vi "FUG-HCN.GetRatedCurrent.vi"(0 "i ref in":refnum<vi>, 2 "Time out":i32, 5 "error in (no error)":errorcluster) -> (14 "i ref out":refnum<vi>, 16 "timed out":bool, 17 "Rated Current{mA}":dbl format="%.2f", 19 "error out":errorcluster)   [LabVIEW 2014, in "FUG-HCN.lvlib"]
doc: "Reads the rated current from the device."
uses:
  FUG-HCN.lvlib
  CSCore/CSSystem/CoreDefs/CoreDefs.error_type.ctl
  CSCore/CSSystem/CoreLib/CoreLib.lvlib
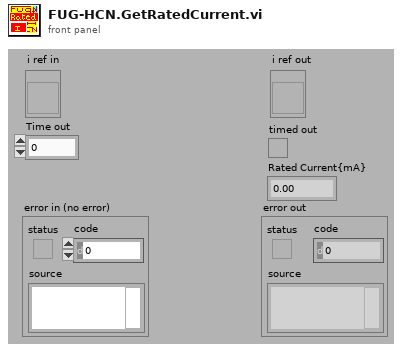
[diagram p1: front panel]
types:
  T1 = cluster{"VISA resource name":refnum<visa-resource-name>, "Gen time out":dbl, "timeout (0)":u32}
  T2 = typedef "CoreDefs.error_type.ctl" = enum16{"no error", "can't load process", "can't unload process", "process does not exist", "can't install process", "can't remove process", "unknown function", "time out", "can't execute function", "duplicate queue name", "super not found", "caller queue invalid", "can't ping process", "unknown error", "VISA Error", "VISA timeout", "GPIB timeout", "GPIB error", "communication error", "data type mismatch", "can't read data from OPC server", "can't write data to OPC server", "OET error", "function not implemented", "process already exists", "invalid Shared Variable name", "error writing Shared Variable", "error reading Shared Variable", "invalid client name", "corrupt database", "unknown class", "call not authorized", "parameter out of range", "OET timeout: can't get data to modify", "invalid queue name", "requested operation incompatible with current state", "event undefined", "event disabled", "state undefined", "caller is not a friend", "EventBuilder: bad eventID", "EventBuilder: no DAQ devices", "a thread must not stop itself", "UNUSED ELEMENT4", "DiscArchiver: eventData incomplete", "DiscArchiver: eventData does not belong to run", "DiscArchiver: can't open file", "DiscArchiver: can't write to file", "DiscArchiver: available disc space low", "can't acquire semaphore", "error reading data from database", "notifier object is not existing", "can't register process", "can't unregister process", "illegal event type", "object disabled", "object already exists", "can't change state", "Instrument not found", "no connection to remote node", "invalid reference", "N/A", "UNUSED ELEMENT 1", "element not found", "illegal TCP/IP connection detected", "object does not exist", "invalid access ID", "unknown CS system", "invalid privilige", "unsupported data type", "unsupported server type", "IO server already exists", "Shared Variable already exists"}
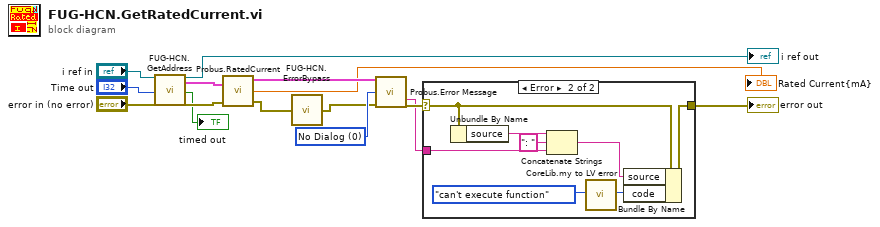
[diagram p0: block diagram]
diagram:
  w5 = 0 items=["No Dialog", "OK Message", "Continue or Stop Message"] ("Type of Dialog (1: OK Msg)")
  n1 = call "FUG-HCN.GetAddress.vi"("i ref in"="i ref in", "Timeout"="Time out", "error in (no error)"="error in (no error)") -> ("i ref out"=→"i ref out":refnum<vi>, "VISA cluster out"=w13:T1, "timed out"=→"timed out":bool, "error out"=w12:errorcluster)  [unwired: 13 in]
  n2 = call "Probus.RatedCurrent.vi"("error in (no error)"=w12, "VISA cluster in"=w13) -> ("error out"=w2:errorcluster, "Rated Current {mA}"=→"Rated Current{mA}":dbl, "VISA cluster out"=w7:T1)  [unwired: 1 in]
  n3 = call "FUG-HCN.ErrorBypass.vi"("error in (no error)"=w2) -> ("error out"=w1:errorcluster)  [unwired: 14 in]
  n4 = call "Probus.Error Message.vi"("Visa Cluster in"=w7, "Type of Dialog (1: OK Msg)"=w5, "error in (no error)"=w1) -> ("Error Message (empty)"=w4:string, "error out"=w6:errorcluster)  [unwired: 8 in, 3 out]
  n5 = case shown="Error" w6 {
    selector: w6 -> [w16 w21]
    tunnel: [w16 w23] -> w10
    tunnel: w4 -> [_ w18]
    frame No Error {
    }
    frame Error {
      n6 = Unbundle By Name(w21) -> ("source"=w20:string)
      n7 = Concatenate Strings(w20, ": " ("string"), w18) -> (w17:string)
      n8 = call "CoreLib.my to LV error.vi"("ErrorTypes"=CoreDefs.error_type."can't execute function") -> ("LV error code"=w22:i32)  [unwired: 17 in, 1 out]
      n9 = Bundle By Name(cluster=w21, "source"=w17, "code"=w22) -> (w23:errorcluster)
    }
  }
  "error out" <- w10
